vi "Move Controls.vi"() -> ()   [LabVIEW 2015, in "DCAF UI Elements.lvlib"]
uses:
  Controls/DCAF UI Elements.lvlib
  Controls/Move One Left.ctl
  Controls/Move One Right.ctl
  Controls/Move All Left.ctl
  Controls/Move All Right.ctl
panel:
  in  "Move All Right":T1
  in  "Move all Left":T2
  in  "Move One Right":T3
  in  "Move One Left":T4
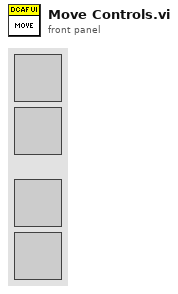
[diagram p1: front panel]
types:
  T1 = typedef "DCAF UI Elements.lvlib/Move All Right.ctl" = bool
  T2 = typedef "DCAF UI Elements.lvlib/Move All Left.ctl" = bool
  T3 = typedef "DCAF UI Elements.lvlib/Move One Right.ctl" = bool
  T4 = typedef "DCAF UI Elements.lvlib/Move One Left.ctl" = bool
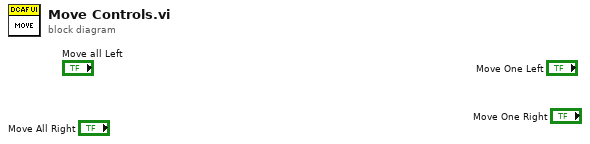
[diagram p0: block diagram]
diagram:
